vi "RenameChannelItem.vi"(9 "TaskConfig":refnum<data-value>, 10 "New Task":string, 11 "Old Task":string) -> ()   [LabVIEW 2025, in "DAQ_Module.lvlib" / "DAQ_Module.lvclass"]
uses:
  DAQ_Module.lvclass
  DAQ_Module.lvclass/DAQ_Module.ctl
  <vilib>/Utility/miscctls.llb/LVMapReplaceAction.ctl
  DAQ_Task_Type.ctl
  DAQ_SampleRateConfig.ctl
  DAQ_HW_Type.ctl
  DAQ_Task_Config.ctl
  DAQ_Config.ctl
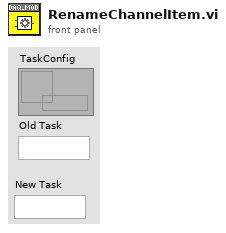
[diagram p1: front panel]
types:
  T1 = typedef "LVMapReplaceAction.ctl" = enum32{"Modify Entry only if found", "Add or Modify Entry", "Delete Entry"}
  T2 = typedef "DAQ_Module.lvlib/DAQ_Module.lvclass/DAQ_Config.ctl" = map{string, T3}
  T3 = typedef "DAQ_Module.lvlib/DAQ_Module.lvclass/DAQ_Task_Config.ctl" = cluster{"Drive":T4, "TaskType":T5, "PhysicalChannels":string, "SampleRateConfiguration":T6, "ChannelConfig":map{string, cluster{"Name":string, "Config":string}}, "Enable":bool, "ShowPanel":bool}
  T4 = typedef "DAQ_Module.lvlib/DAQ_Module.lvclass/DAQ_HW_Type.ctl" = enum16{"NI_DAQmx", "Simulated_DAQ"}
  T5 = typedef "DAQ_Module.lvlib/DAQ_Module.lvclass/DAQ_Task_Type.ctl" = enum16{"AI", "Linear", "Angular", "AO"}
  T6 = typedef "DAQ_Module.lvlib/DAQ_Module.lvclass/DAQ_SampleRateConfig.ctl" = cluster{"SampleRate":dbl, "SamplesPerChannel":u32, "SamplesPerRead":i32, "SampleMode":i32, "Clock Source":string}
  T7 = map{string, cluster{"Name":string, "Config":string}}
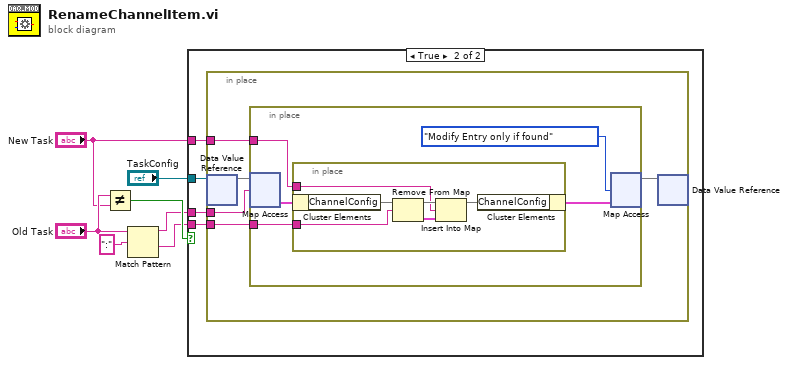
[diagram p0: block diagram]
diagram:
  n1 = Not Equal?(x="Old Task", y="New Task") -> (x != y?=w6:bool)
  n2 = Match Pattern(string="Old Task", regular expression=":") -> (before substring=w3:string, after substring=w2:string)  [unwired: 1 in, 2 out]
  n3 = case shown="True" w6 {
    tunnel: "TaskConfig" -> [_ w11]
    tunnel: w3 -> [_ w10]
    tunnel: w2 -> [_ w9]
    tunnel: "New Task" -> [_ w8]
    frame False {
    }
    frame True {
      n4 = in-place {
        in-place-border: w10 -> [w15]
        in-place-border: w9 -> [w13]
        in-place-border: w8 -> [w12]
        n5 = in-place-dvr #1(w11) -> (w16:T2)  [unwired: 1 out]
        n6 = in-place {
          in-place-border: w13 -> [w18]
          in-place-border: w12 -> [w17]
          n7 = in-place-map #2(w16, w15) -> (w20:T3)  [unwired: 1 in, 1 out]
          n8 = in-place {
            in-place-border: w18 -> [w26]
            in-place-border: w17 -> [w24]
            n9 = in-place-cluster #3(w20) -> ("ChannelConfig"=w27:T7)
            n10 = Remove From Map(10:w26, 11:w27) -> (1:w23:cluster{"Name":string, "Config":string}, 3:w25:T7)  [unwired: 1 out]
            n11 = Insert Into Map(map in=w25, key=w24, value=w23) -> (map out=w22:T7)  [unwired: 2 out]
            n12 = in-place-cluster #3("ChannelConfig"=w22) -> (w19:T3)
          }
          n13 = in-place-map #2(w19, LVMapReplaceAction."Modify Entry only if found" ("action")) -> (w14:T2)  [unwired: 2 out]
        }
        n14 = in-place-dvr #1(w14) -> ()  [unwired: 2 out]
      }
    }
  }
